vi "Init LaunchPad.vi"(8 "error in":errorcluster, 10 "Baud Rate (9600)":u32=9600, 11 "VISA resource":refnum<visa-resource-name>) -> (0 "error out":errorcluster, 3 "VISA resource name out":refnum<visa-resource-name>)   [LabVIEW 2015]
doc: "Initializes a connection to an Arduino running the LabVIEW Interface for Arduino sketch.\n\nNote: The baud rate specified must match the baud rate defined by DEFAULTBAUDRATE in the Arduino firmware.\n\nNote: The Bytes Per Packet input must match the COMMANDLENGTH specified in the Arduino firmware."
uses:
  <vilib>/Instr/_visa.llb/VISA Configure Serial Port (Instr).vi
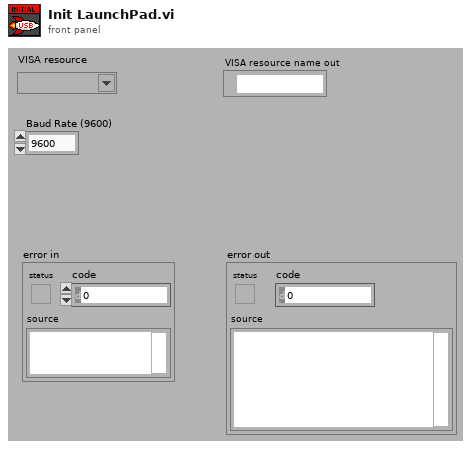
[diagram p1: front panel]
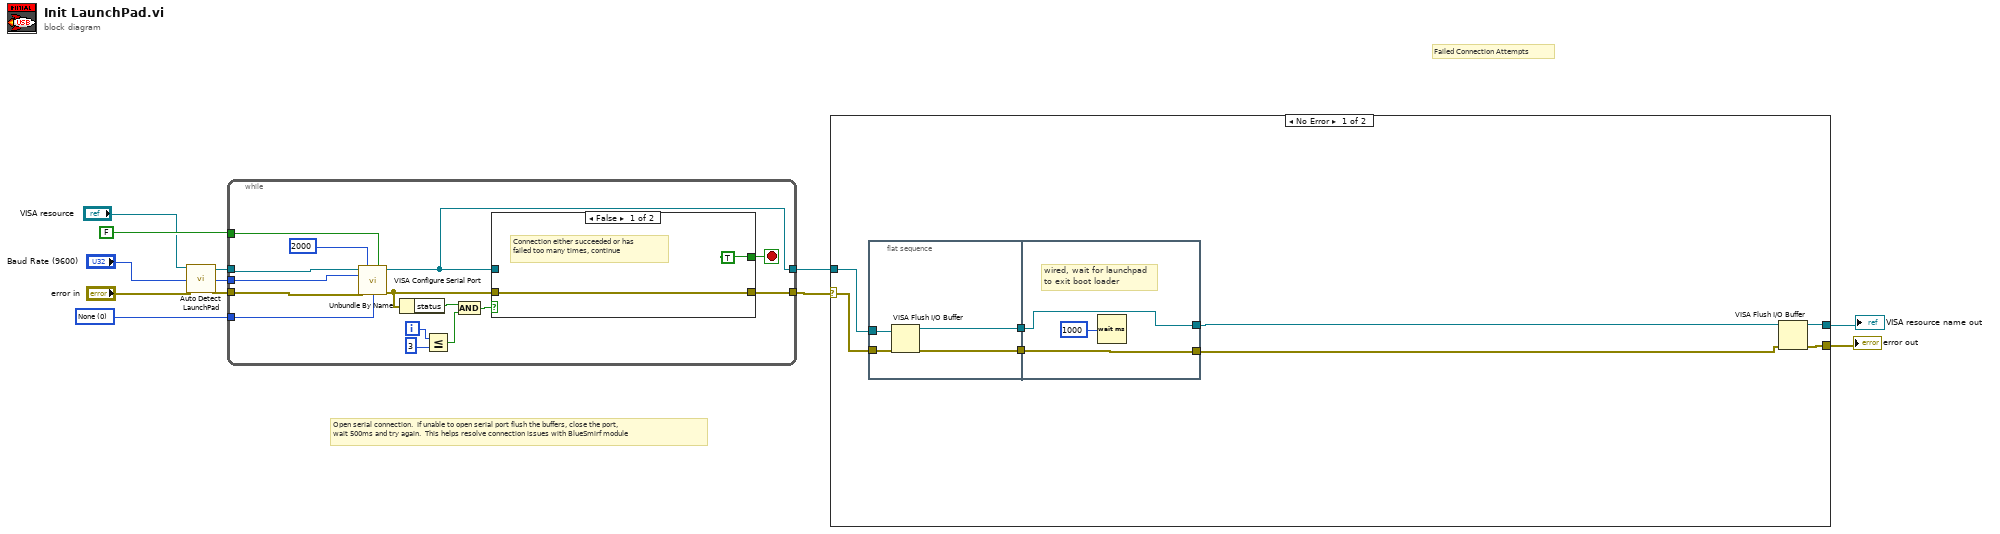
[diagram p0: block diagram]
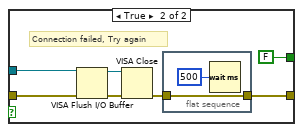
[diagram p3: hidden frame]
diagram:
  w11 = u16 0 items=["None", "XON/XOFF", "RTS/CTS", "XON/XOFF & RTS/CTS", "DTR/DSR", "XON/XOFF & DTR/DSR"] ("flow control (0:none)")
  # "Failed Connection Attempts"
  # "Open serial connection.  If unable to open serial port flush the buffers, close the port,\nwait 500ms and try again.  This helps resolve connection issues with BlueSmirf module"
  n1 = call "Auto Detect LaunchPad.vi"("Visa Resource"="VISA resource", "error in (no error)"="error in") -> ("VISA resource"=w8:refnum<visa-resource-name>, "error out"=w5:errorcluster)  [unwired: 12 in]
  n2 = while {
    tunnel: w11 -> [w26]
    tunnel: FALSE ("Enable Termination\nChar (T)") -> [w25]
    tunnel: "Baud Rate (9600)" -> [w24]
    tunnel: w8 -> [w13]
    tunnel: [w17] -> w1
    tunnel: [w15] -> w3
    tunnel: w5 -> [w12]
    i -> [w22]
    stop <- w16 stop-if-true
    n3 = call-poly "VISA Configure Serial Port"("VISA resource name"=w13, "timeout (10sec)"=u32 2000, "Enable Termination\nChar (T)"=w25, "baud rate (9600)"=w24, "error in (no error)"=w12, "flow control (0:none)"=w26) -> ("VISA resource name out"=w15:refnum<visa-resource-name>, "error out"=w18:errorcluster)  [unwired: 8 in]
    n4 = Unbundle By Name(w18) -> ("status"=w20:bool)
    n5 = Less Or Equal?(x=w22, y=3) -> (x <= y?=w21:bool)
    n6 = And(x=w20, y=w21) -> (x .and. y?=w19:bool)
    n7 = case shown="False" w19 {
      tunnel: w18 -> [w28 w31]
      tunnel: [w28 w30] -> w17
      tunnel: [TRUE FALSE] -> w16
      tunnel: w15 -> [_ w34]
      frame False {
        # "Connection either succeeded or has \nfailed too many times, continue"
      }
      frame True {
        # "Connection failed, Try again"
        n8 = VISA Flush I/O Buffer(VISA resource name=w34, error in (no error)=w31) -> (VISA resource name out=w33:refnum<visa-resource-name>, error out=w32:errorcluster)  [unwired: 1 in]
        n9 = VISA Close(VISA resource name=w33, error in (no error)=w32) -> (error out=w29:errorcluster)
        n10 = flat-sequence {
          tunnel: [w36] -> w30
          tunnel: w29 -> [w36]
          frame #0 {
            n11 = Wait (ms)(milliseconds to wait=u32 500) -> ()  [unwired: 1 out]
          }
        }
      }
    }
  }
  n12 = case shown="No Error" w1 {
    selector: w1 -> [w42 w53]
    tunnel: [w41 w53] -> w4
    tunnel: w3 -> [w44 w54]
    tunnel: [w40 w54] -> w2
    frame No Error {
      n13 = flat-sequence {
        tunnel: [w48] -> w45
        tunnel: w42 -> [w49]
        tunnel: w44 -> [w47]
        tunnel: [w46] -> w43
        tunnel: [w52] -> w39
        tunnel: w45 -> [w52]
        tunnel: w43 -> [w50]
        tunnel: [w50] -> w38
        frame #0 {
          n14 = VISA Flush I/O Buffer(VISA resource name=w47, error in (no error)=w49) -> (VISA resource name out=w46:refnum<visa-resource-name>, error out=w48:errorcluster)  [unwired: 1 in]
        }
        frame #1 {
          # "wired, wait for launchpad \nto exit boot loader"
          n15 = Wait (ms)(milliseconds to wait=u32 1000) -> ()  [unwired: 1 out]
        }
      }
      n16 = VISA Flush I/O Buffer(VISA resource name=w38, error in (no error)=w39) -> (VISA resource name out=w40:refnum<visa-resource-name>, error out=w41:errorcluster)  [unwired: 1 in]
    }
    frame Error {
    }
  }
  "VISA resource name out" <- w2
  "error out" <- w4
